vi "Exit.vi"(8 "error in (no error)":errorcluster, 11 "Running in":refnum<class "Guiding.lvclass">) -> (0 "error out":errorcluster, 3 "Running out":refnum<class "Guiding.lvclass">)   [LabVIEW 2014, in "States.lvlib" / "Guiding.lvclass"]
doc: "This override sends a Stop Acquisition message to the Process Actor. It also sends a Log Event message to the UI, with the string containing \"Exiting Running State\", the average value of the data stream, and the total number of elements of the steam as its payload."
uses:
  Guiding.lvclass
  <vilib>/ActorFramework/Message Enqueuer/Message Enqueuer.lvclass/Message Enqueuer.ctl
  <vilib>/ActorFramework/Message Enqueuer/Enqueue.vi
  <vilib>/ActorFramework/Message Priority Queue/Priority Enqueue.vi
  Process State/CoordinatorState.lvclass
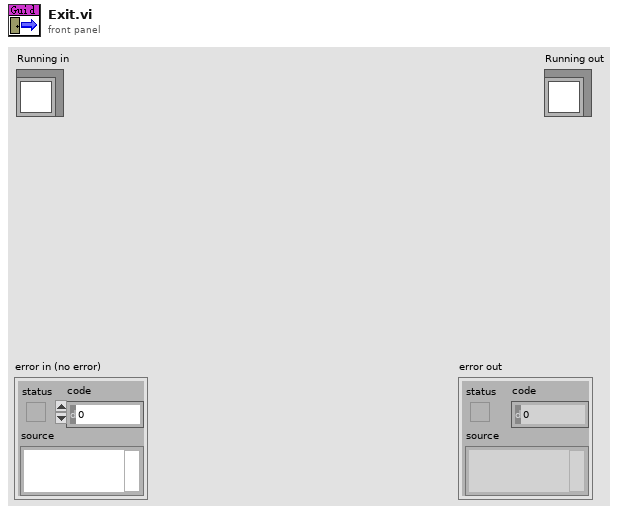
[diagram p1: front panel]
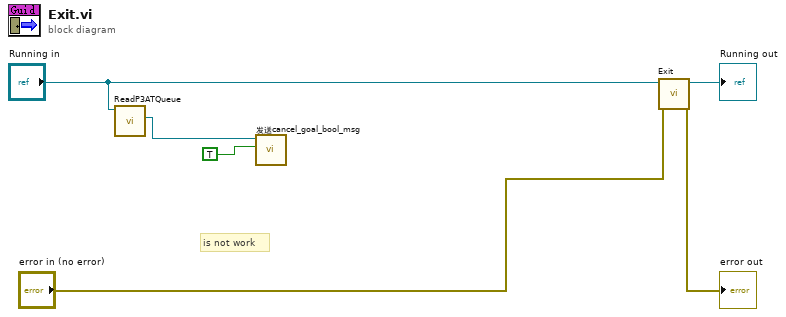
[diagram p0: block diagram]
diagram:
  # "is not work"
  n1 = call-dynamic "ReadP3ATQueue.vi"("CoordinatorState输入"="Running in") -> ("操作者框架:消息待入队列"=w2:refnum<class "Message Enqueuer.lvclass">)  [unwired: 8 in, 2 out]
  n2 = call "发送cancel_goal_bool_msg.vi"("值(信号)"=TRUE, "消息待入队列"=w2) -> ()  [unwired: 8 in, 2 out]
  n3 = call-parent "Exit.vi"("error in (no error)"="error in (no error)", "Old State"="Running in") -> ("error out"=→"error out":errorcluster, "New State"=→"Running out":refnum<class "Guiding.lvclass">)  [unwired: 8 in]
